vi "Gel Tugging Force Mode_Data Logger v16.20 DIC.vi"() -> ()   [LabVIEW 2015]
uses:
  <vilib>/Utility/error.llb/DialogType.ctl
  <vilib>/DAQmx/read.llb/DAQmx Read (Analog 2D DBL NChan NSamp).vi
  <vilib>/DAQmx/create/channels.llb/DAQmx Create Channel (AI-Voltage-Basic).vi
  <vilib>/DAQmx/configure/timing.llb/DAQmx Timing (Sample Clock).vi
  <vilib>/DAQmx/configure/trigger.llb/DAQmx Start Trigger (Digital Edge).vi
  <vilib>/DAQmx/miscellaneous.llb/DAQmx Fill In Error Info.vi
  <vilib>/Utility/file.llb/Write Delimited Spreadsheet (DBL).vi
  <resource>/objmgr/daqmx.rc
  <resource>/objmgr/ni.dex.rc
panel:
  in  "Filename: 2":string="R1"
  out "Loop Index":u64
  in  "Working Directory":path=path "F:/EDAC_Experiments" caption="Path"
  out "Current Plot (V)":dbl[](graph)
  out "Exposure Plot (V)":dbl[](graph)
  out "Flux Plot (V)":dbl[](graph)
  in  "Start Manual Trigger Button":bool
  in  "Trigger Type?":bool=TRUE
  in  "Notes:":string="0.75 mg/mL type I collagen gel (initial ~7.4 pH) placed in a humified incubator @ 37°C/5%CO2, Prepared on 2021-12-20\nNOT Covered with 2.6mM EDAC + 0.1M MES (pH~ 6.0) solution for 30 minutes. 1X DPBS Wash as a negative \"Treatment\"\n18-mm diameter Sylgard 184 1:10 mixture\nSylgard Mold removed after polymerization, before coating and testing.\nWashed the gel before adding the red beads with clean milliQ water\n~ 170 µL of collagen gel mix  => ~ 330 mm \n~ 350 µL of 0.09 µL M450 bead/mL was used to coat the gel until setting. Prepare as per manufacturer protocol.\n~ 350 µL of  8 µL Fluorosphere beads/mL Milli-Q water were used to coat the gel for 30 seconds\nPreconditioning of gel: at least 9 full cycles of ON/OFF with the needle tip at the start location.\nStock rat-tail type I collagen: 3.04 mg/mL. Corning. REF: 354236. Lot #:1077003\nFluoSpheres™ Carboxylate-Modified Microspheres, 0.5 µm, red fluorescent (580/605), 2% solids. REF: F8812. Lot: 2291412.\nDynabeads™ M-450 Tosylactivated 4.5 µm superparamagnetic beads containing surface tosyl groups. REF: 14013. Lot: 00789712."
  out "Total Ramp \nTime (ms)":i16
  out "# Ramp\nSteps":i16
  in  "Fluoro Beads\nDiameter (Micron)":dbl=0.5 format="%#.1g"
  in  "Tip Initial XY Separation\n (micron)":dbl=17.0
  in  "Frame Scale \n(micron/pixel)":dbl=0.24281
  in  "Gel Thickness\n(Micron)":dbl=345.0
  in  "Fluoro Beads \nZ-Level\n(Micron)":dbl
  in  "Magnetic \nBead Z-Level\n(Micron)":dbl
  in  "Tip Z-level Above Gel Surface (micron)":dbl=10.0
  out "Digital Trigger":bool
  out "Flux On\n Setpoint (Gs)":dbl=2.4945191 format="%.3g"
  out "Column 4":string="Flux Sensor (V)"
  out "Column 3":string="Flux Sensor (V)"
  out "Column 1":string="Flux Sensor (V)"
  out "Column 2":string="Flux Sensor (V)"
  in  "Temperature\n(ºC)":dbl=24.8
  out "Ready?":bool
  in  "?":bool
  in  "Relative \nHumidity (%)":dbl=22.0
  out "Magnetic Flux Sensor\n Sensitivity (V/Gs)":dbl=2.4945191 format="%#_8g"
  in  "Magnetic Bead\nDiameter (Micron)":dbl=4.5 format="%#.1g"
  in  "Needle\n Inclination \nAngle (º)":dbl=25.0
  out "Data Points":u64
  out "Cycles":i16
  out "Downloading\nData":bool
  out "Magnetic Flux Sensor\n Zero, Crude Mean (V)":dbl=2.4945191 format="%.6g"
  in  "Filename:":string="S20211220.12mm.1_0.75mgmL_37C-B1.348um-NoEDC.CO2"
  # "For Gel Tugging Experiments v16.20-DIC Part"
  # "Verify Data Further with  \"Gel Tugging Force Mode_Data Reduction v16.00.vi\" or \"ReadSensorData.m\" in MATLAB"
  # "Step 1: Enter:"
  # "-DIC-"
  # ".dat"
  # "&"
  # "_Notes.txt"
  # "Manual"
  # "Automatic"
  # "Step 2: Click TRGR or Run Macro in Nikon Elements"
  # "datapoints downloaded"
  # "out of"
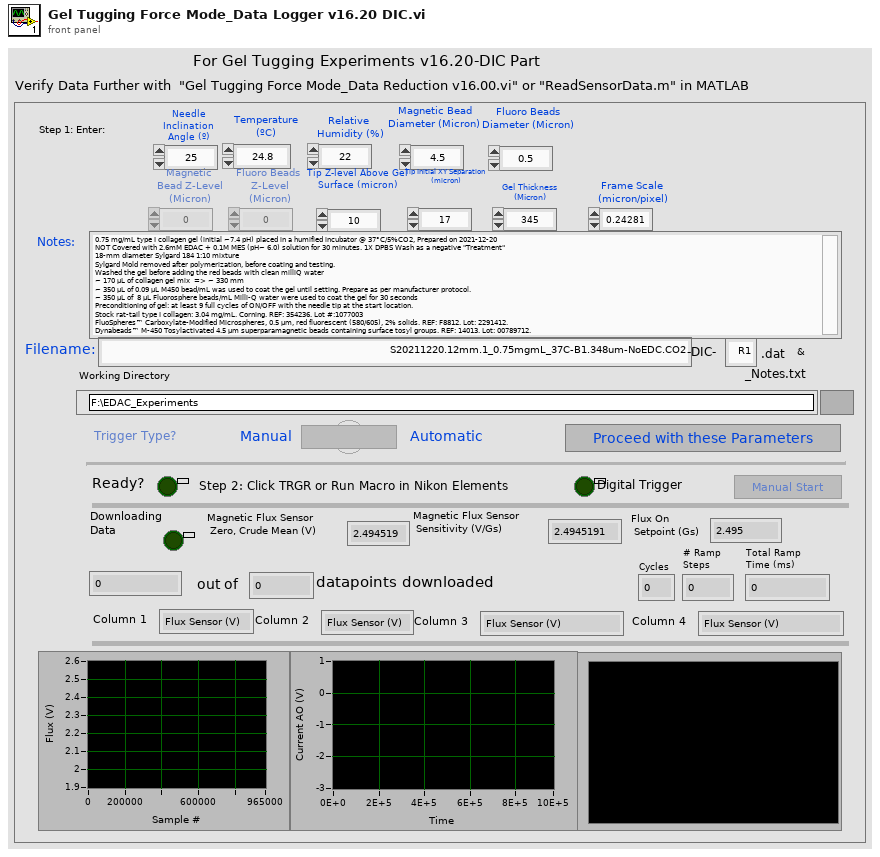
[diagram p1: front panel]
types:
  T1 = enum8{"Enabled", "Disabled", "Disabled and Grayed Out"}
  T2 = typedef "DialogType.ctl" = u16
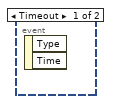
[diagram p2: hidden frame]
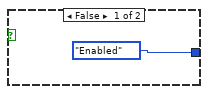
[diagram p3: hidden frame]
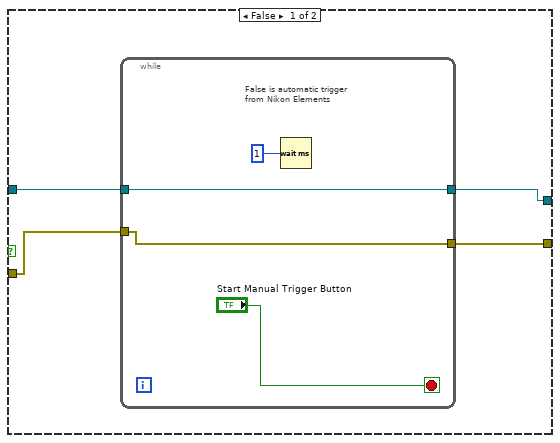
[diagram p4: hidden frame]
diagram:
  # "Modified from v15.00 by #Waddah #Moghram on 12/18/2018 and thereafter.\n1. Added a note section that will be in a file with the same note, but add \"notes\" to it. \n2. Tip -> Magnetic Bead. Magnetic Bead -> Fluorobeads. Fluoro beads -> Tip z-level. Headers were corrected 12/20/2018\n \nModified from v11.00 by #Waddah #Moghram on 5/4/2018 and thereafter:\n1. Updated the header to include gel-related information such as z-levels for the tip, bead, and thickness; gel thickness.\n2. Changed output file extension to *.dat\n3. Added a few other headers. Updated Ramp Step Information 11/28/2018\n\nModified from v10.00 by #Waddah #Moghram on 4/26/2018:\n1. This program will get the digital trigger from Nikon Elements. Then it will forward it to the control sequence VI on the slave DAQ for real-time sequence. This is a roundabout way to deal with the issue of ground loop problems.\n\nModified from v8.00 and later by #Waddah #Moghram on 4/4/2018 \n2. Just add an extra Row...with Null Flux Corrective just for the record. Did not mess with anything previously\n2. \"Flux Observed Zero\" renamed to \"Null Flux Observed\"\n3. \"AO Signal\" is replaced back to \"Camera Exposure (V)\"\n4. Added Labels \"Rows\" to the Header to keep track\n5. Updated Samples read per loop from 400 to 40000 4/1/2018\n6. Added Headers for Gel properties\n\nModified from v7.40 by #Waddah #Moghram on 1/4/2018\n1. Remove Step 0: Recording temperature with thermocouple. Thermocouple reading is not reliable, whether is the one built into labVIEW or the handheld one. Enter the value read by the Digital Thermometer along with relative humidity readings.\n2. Added an extra row to store both sets of PIDs for ON/OFF. \n3. Modified Tabbing Order on 3/4/2018\n4. Added Columns Display at front panel 3/18/2018\n\nModified from v7.30 by #Waddah #Moghram on 12/23/2017\n1. Added event close loop to make the Data Logger Running False if user closes it abruptly. \nNote: Aborting event is not included. Avoid aborting if possible.\n2. corrected total number of data points to allow for more than 2 seconds 1/4/2018 by #WIM\n\nModified from v7.00 by #Waddah #Moghram on 12/21/2017\n1. Reduce Thermocouple time to 1 \n2. Added another Text to record room temperature manual. But be consistent.\n\nModified from v6.00 by #Waddah #Moghram on 12/18/2017\n1. Added Relative Humidity Entry instead of \"Dummy Variable Entry in the Header.\" This value is to be entered from the reading of Relative Humidity\\\n2. Added Thermocouple measurement VI into this one. Average and storage into Data Logger for future purposes. \n\nModified from v5.22 by #Waddah #Moghram on 12/05/2017\n1. Added Entry for Magnetic Sensor Sensitivity\n2. Added Precisions for Header Values\n\nModified from v.4.00 by #Waddah #Moghram on 8/9/2017\n\nModified from v.3.80 by #Waddah #Moghram on 8/7/2017\n*Current Dialog boxes. Use Stacked sequences. Cleaned up v.3.80\n*Included Post  & Pre-wave Periods in Data Collection\n\nModified by #Waddah #Moghram on 8/7/2017\n*Include PID Parameters in the file\n*Modified headers of columns to be able to be extracted from MATLAB\n*Network stream loop is cleaned up \n*Removed Data Logging Time. Whatever it it takes to download the entire stream.\n*works with local single process FIFO\n\nDigital Input (Trigger)\n1. Dev3/PFI0 is connected internally in the DAQ-1/Master Connecter block. It is also wired up to DAQ-2/Slave Connector Block\n\nModifications from previous edition:\n1. Removed AI1 & AI2 to see if instability is due to a ground loop.\n\nNote: Sampling rate for Data Logger is 10,000 Samples/Second"
  n1 = flat-sequence {
    tunnel: [w18] -> w2
    tunnel: [w28] -> w12
    tunnel: [w29] -> w11
    tunnel: w2 -> [w25]
    tunnel: [w25] -> w1
    tunnel: w12 -> [w42]
    tunnel: w11 -> [w41]
    tunnel: [w43] -> w7
    tunnel: [w44] -> w3
    tunnel: w1 -> [w40]
    tunnel: [w225] -> w8
    tunnel: w7 -> [w158]
    tunnel: [w158] -> w6
    tunnel: [w288] -> w5
    tunnel: [w164] -> w4
    tunnel: w3 -> [w288]
    tunnel: w8 -> [w302]
    tunnel: w6 -> [w307]
    tunnel: [w296] -> w10
    tunnel: w5 -> [w306]
    tunnel: [w301] -> w9
    tunnel: w4 -> [w315]
    tunnel: w10 -> [w382]
    tunnel: w9 -> [w381]
    frame #0 {
      w16 = FALSE ("Data Download")
      (unwired) "1. OPEN the PID Control VI & Follow Instructions **if you have not done so already**.\n2. Click OK to begin temperature measurement & ENTER other variables afterwards.\n3. RUN the macro (if a macro is used). Otherwise, CLICK  \"TRGR\" button in Nikon Elements to initiate Fast Timelapse Image Capture, Data Acquisition, and PID-Controlled Sequence."
      # "Clear Graphs"
      # "Reset the Data Download"
      n2 = property on="Flux Plot (V)" class="WFGraph (strict)"("Value"=dbl[] [] ("Flux Plot (V)")) -> ()  [unwired: 2 in, 2 out]
      n3 = property on="Current Plot (V)" class="WFGraph (strict)"("Value"=dbl[] [] ("Current Plot (V)")) -> ()  [unwired: 2 in, 2 out]
      n4 = property on="Exposure Plot (V)" class="WFGraph (strict)"("Value"=dbl[] [] ("Exposure Plot (V)")) -> ()  [unwired: 2 in, 2 out]
      n5 = shared-variable "NI-GenericDesktopPC-3A84958E\\Kopco PS Project Target Variables Library.lvlib\\Data Download"(w16) -> ()  [unwired: 1 in, 1 out]
      n6 = shared-variable "NI-GenericDesktopPC-3A84958E\\Kopco PS Project Target Variables Library.lvlib\\Data Logger Running"(TRUE ("Data Logger Running")) -> ()  [unwired: 1 in, 1 out]
      n7 = shared-variable "NI-GenericDesktopPC-3A84958E\\Kopco PS Project Target Variables Library.lvlib\\Temperature Measured"(w16) -> ()  [unwired: 1 in, 1 out]
      n8 = shared-variable "NI-GenericDesktopPC-3A84958E\\Kopco PS Project Target Variables Library.lvlib\\Experiment Settings Entered"(w16) -> ()  [unwired: 1 in, 1 out]
      n9 = shared-variable "NI-GenericDesktopPC-3A84958E\\Kopco PS Project Target Variables Library.lvlib\\Digital Trigger"(w16) -> ()  [unwired: 1 in, 1 out]
    }
    frame #1 {
      # "Gives a pause to adjust the values before confirmation"
      # "Bound to \"Experiment Settings Entered\"\nglobal shared variable."
      n10 = while {
        tunnel: ["?"] -> w19
        tunnel: ["Trigger Type?"] -> w18
        stop <- "?" stop-if-true
        n11 = case shown="True" "Trigger Type?" {
          tunnel: [T1."Enabled" ("Disabled") T1."Disabled and Grayed Out" ("Disabled")] -> w22
          frame False {
          }
          frame True {
          }
        }
        n12 = property on="Start Manual Trigger Button" class="Bool"("Disabled"=w22) -> ()  [unwired: 2 in, 2 out]
      }
      n13 = shared-variable "NI-GenericDesktopPC-3A84958E\\Kopco PS Project Target Variables Library.lvlib\\Experiment Settings Entered"(w19) -> ()  [unwired: 1 in, 1 out]
    }
    frame #2 {
      w26 = 30000.0  # AI Frequency
      w30 = 10106 items=["Default"=-1, "RSE"=10083, "NRSE"=10078, "Differential"=10106, "Pseudodifferential"=12529] ("input terminal configuration")
      w31 = 10123 items=["Finite Samples"=10178, "Continuous Samples"=10123] ("sample mode")
      # "Configuring Analog Inputs (AIs)\n3. Dev2/AI5 is connected to \"RAW\" Magnetic Flux Sensor\n4. Dev2/AI6 is connected to \"Current Senssor (1A/V)\"\n5. Dev2/AI7 is connected to Camera Exposure Signal (\"Out 4\" on sCMOS Camera)"
      # "As of 8/3/2017. This is \njust to initiate digital trigger.\nNo data is collected via master DAQ"
      n14 = call-poly <vilib>:"DAQmx Create Virtual Channel.vi"("maximum value"=10.0, "minimum value"=-10.0, "input terminal configuration"=w30, "physical channels"="Dev3/ai3") -> ("task out"=w33:refnum<k21>, "error out"=w32:errorcluster)  [unwired: 10 in]
      n15 = call-poly <vilib>:"DAQmx Timing.vi"("task/channels in"=w33, "sample mode"=w31, "rate"=w26, "source"=tag "OnboardClock" ("Sample Clock Source"), "error in"=w32) -> ("task out"=w34:refnum<k21>, "error out"=w35:errorcluster)  [unwired: 9 in]
      n16 = call <vilib>:"DAQmx Configure Input Buffer.vi"("task/channels in"=w34, "buffer size (in samples per channel)"=200000, "error in"=w35) -> ("task out"=w28:refnum<k21>, "error out"=w29:errorcluster)  [unwired: 11 in]
    }
    frame #3 {
      n17 = case shown="True" w40 {
        tunnel: [w48 w66] -> w45
        tunnel: w41 -> [w49 w58]
        tunnel: [w51 w57] -> w46
        tunnel: w42 -> [w50 w56]
        frame False {
          n18 = while {
            tunnel: [w54] -> w51
            tunnel: w50 -> [w54]
            tunnel: w49 -> [w53]
            tunnel: [w53] -> w48
            stop <- "Start Manual Trigger Button" stop-if-true
            # "False is automatic trigger \nfrom Nikon Elements"
            n19 = Wait (ms)(milliseconds to wait=u32 1) -> ()  [unwired: 1 out]
          }
        }
        frame True {
          w59 = 10280 items=["Rising"=10280, "Falling"=10171] ("edge")
          # "True is automatic trigger \nfrom Nikon Elements"
          # "Waiting for Digital Trigger (\"TRGR\") from Nikon Element\nOr Macro that has a digital trigger"
          n20 = call-poly <vilib>:"DAQmx Trigger.vi"("task/channels in"=w56, "source"=tag "/Dev3/PFI0", "edge"=w59, "error in"=w58) -> ("task out"=w61:refnum<k21>, "error out"=w63:errorcluster)  [unwired: 10 in]
          n21 = property class="DAQmx Trigger"(reference=w61, error in=w63, "Start.DigEdge.DigFltr.MinPulseWidth"=1e-06) -> (reference out=w62:refnum<k21>, error out=w64:errorcluster)
          n22 = call <vilib>:"DAQmx Start Task.vi"("task/channels in"=w62, "error in"=w64) -> ("task out"=w57:refnum<k21>, "error out"=w66:errorcluster)  [unwired: 12 in]
        }
      }
      n23 = while "Just a one-item loop for to start the digital trigger" {
        tunnel: w45 -> [w73]
        tunnel: w46 -> [w72]
        tunnel: [w71] -> w44
        tunnel: [w70] -> w43
        tunnel: [w67] -> w47
        i -> [w69]
        stop <- w67 stop-if-true
        w75 = -1.0  # timeout
        # "Added on 4/24/2018. Digital Trigger to be transferred to \nRT control sequence VI"
        n24 = Equal?(x=1, y=w69) -> (x = y?=w67:bool)
        n25 = call-poly <vilib>:"DAQmx Read.vi"("task/channels in"=w72, "number of samples per channel"=1, "timeout"=w75, "error in"=w73) -> ("task out"=w71:refnum<k21>, "error out"=w70:errorcluster)  [unwired: 9 in, 1 out]
        n26 = Unbundle By Name(w70) -> ()  [unwired: 1 out]
      }
      n27 = shared-variable "NI-GenericDesktopPC-3A84958E\\Kopco PS Project Target Variables Library.lvlib\\Digital Trigger"(w47) -> ()  [unwired: 1 in, 1 out]
    }
    frame #4 {
      w114 = 0.0  # number
      w130 = "\t"
      w132 = "\t"
      w155 = "\t"
      w154 = "\t"
      w169 = "\t"
      w168 = "\t"
      (unwired) "AO Signal (V)" ("string")
      w189 = "\t"
      w187 = "\t"
      w215 = "\t"
      w213 = "\t"
      w274 = "\t"
      w272 = "\t"
      w240 = "\t"
      w238 = "\t"
      w175 = "Current AO (V)" ("string")
      w254 = "\t"
      w257 = "\t"
      w166 = "Camera Exposure TTL (V)" ("string")
      w251 = "\t"
      w174 = "Current Sensor (V or A)" ("string")
      w250 = "Flux Sensor (V)" ("string")
      # "Added on 3/17/2018\nfor mini DeGauss & \ntuning experiments. \nModify controller Program accordingly.\n4/4/2018. Back to Camera Exposure"
      # "Added on 3/17/2018\nfor mini DeGauss & \ntuning experiments. \nModify controller Program accordingly.\n4/4/2018. Back to Camera Exposure"
      # "Step Duration is changed to \nSampling Rate, 1/5/2018 by WIM"
      # "Sampling Rate (samples/sec)"
      # "Removed (%) on 12/20/2017 @ 6:58 PM.\nIt should not be % since it is alreayd in decimal. Otherwise, it is %"
      # "Changed from (mV/Gs) to (V/Gs) on 7/18/2017"
      # "Modified on 7/19/2017 to Including Sampling Frequency \ninstead of Sampling Rate to minimize round off Error"
      # "3rd Line Header"
      # "Magentic Sensor Sensitivity"
      n28 = shared-variable "NI-GenericDesktopPC-3A84958E\\Kopco PS Project Target Variables Library.lvlib\\Flux Setpoint ON Gs Relative"() -> (w161:dbl)  [unwired: 1 in, 1 out]
      "Flux On\n Setpoint (Gs)" <- w161
      n29 = shared-variable "NI-GenericDesktopPC-3A84958E\\Kopco PS Project Target Variables Library.lvlib\\Null Flux Pre Period"() -> (w285:dbl)  [unwired: 1 in, 1 out]
      n30 = shared-variable "NI-GenericDesktopPC-3A84958E\\Kopco PS Project Target Variables Library.lvlib\\Temperature"("Temperature\n(ºC)") -> ()  [unwired: 1 in, 1 out]
      n31 = shared-variable "NI-GenericDesktopPC-3A84958E\\Kopco PS Project Target Variables Library.lvlib\\Zero Flux Observed GS"() -> (w284:dbl)  [unwired: 1 in, 1 out]
      n32 = shared-variable "NI-GenericDesktopPC-3A84958E\\Kopco PS Project Target Variables Library.lvlib\\Null Flux Post Period"() -> (w286:dbl)  [unwired: 1 in, 1 out]
      n33 = shared-variable "NI-GenericDesktopPC-3A84958E\\Kopco PS Project Target Variables Library.lvlib\\MagneticBeadDiameterMicron"("Magnetic Bead\nDiameter (Micron)") -> ()  [unwired: 1 in, 1 out]
      n34 = shared-variable "NI-GenericDesktopPC-3A84958E\\Kopco PS Project Target Variables Library.lvlib\\PID Parameters ON"() -> (w227:dbl[])  [unwired: 1 in, 1 out]
      n35 = shared-variable "NI-GenericDesktopPC-3A84958E\\Kopco PS Project Target Variables Library.lvlib\\Sensor Sensitivity Core"() -> (w210:dbl)  [unwired: 1 in, 1 out]
      "Magnetic Flux Sensor\n Sensitivity (V/Gs)" <- w210
      n36 = shared-variable "NI-GenericDesktopPC-3A84958E\\Kopco PS Project Target Variables Library.lvlib\\NeedleInclinationAngle"("Needle\n Inclination \nAngle (º)") -> ()  [unwired: 1 in, 1 out]
      n37 = shared-variable "NI-GenericDesktopPC-3A84958E\\Kopco PS Project Target Variables Library.lvlib\\RelativeHumidity"("Relative \nHumidity (%)") -> ()  [unwired: 1 in, 1 out]
      n38 = shared-variable "NI-GenericDesktopPC-3A84958E\\Kopco PS Project Target Variables Library.lvlib\\Zero Flux Calibrated Core"() -> (w258:dbl)  [unwired: 1 in, 1 out]
      "Magnetic Flux Sensor\n Zero, Crude Mean (V)" <- w258
      n39 = Index Array(array=w227, index=3) -> (element=w287:dbl)
      n40 = Index Array(array=w227, index=4) -> (element=w164:dbl)
      n41 = Index Array(array=w227, index=2) -> (element=w231:dbl)
      n42 = Number To Fractional String "Flux ON Relative Setpoint (Gs)"(number=w161) -> (F-format string=w279:string)  [unwired: 3 in]
      n43 = Number To Fractional String "Flux Observed Zero (Gs)"(number=w284) -> (F-format string=w278:string)  [unwired: 3 in]
      n44 = Index Array(array=w227, index=1) -> (element=w234:dbl)
      n45 = Index Array(array=w227, index=0) -> (element=w236:dbl)
      n46 = Number To Fractional String "Pre- Zero Interval (s)"(number=w285) -> (F-format string=w277:string)  [unwired: 3 in]
      n47 = Number To Fractional String "Post- Zero Interval (s)"(number=w286) -> (F-format string=w273:string)  [unwired: 3 in]
      n48 = Divide(x="Relative \nHumidity (%)", y=100.0) -> (x/y=w204:dbl)
      n49 = shared-variable "NI-GenericDesktopPC-3A84958E\\Kopco PS Project Target Variables Library.lvlib\\Cycles"() -> (w270:i16)  [unwired: 1 in, 1 out]
      n50 = shared-variable "NI-GenericDesktopPC-3A84958E\\Kopco PS Project Target Variables Library.lvlib\\PID Parameters OFF"() -> (w173:dbl[])  [unwired: 1 in, 1 out]
      n51 = Number To Fractional String "Proportional Gain (K_c)"(number=w236) -> (F-format string=w246:string)  [unwired: 3 in]
      n52 = Number To Exponential String "Integral Time (T_i, min)"(number=w234) -> (E-format string=w245:string)  [unwired: 3 in]
      n53 = shared-variable "NI-GenericDesktopPC-3A84958E\\Kopco PS Project Target Variables Library.lvlib\\Needle Used"() -> (w176:i8)  [unwired: 1 in, 1 out]
      n54 = Number To Fractional String "Magnetic Sensor Mean, Crude"(number=w258, precision (6)=i16 6) -> (F-format string=w261:string)  [unwired: 2 in]
      n55 = Number To Exponential String "Derivative Time (T_d, min)"(number=w231) -> (E-format string=w244:string)  [unwired: 3 in]
      n56 = Number To Fractional String "Samples Pushed to PID at a time"(number=w287, precision (6)=i16 0) -> (F-format string=w239:string)  [unwired: 2 in]
      n57 = Number To Fractional String "Number of Cycles"(number=w270, precision (6)=i16 0 ("width (-)")) -> (F-format string=w259:string)  [unwired: 2 in]
      n58 = Number To Fractional String "Sampling Rate (Samples/Sec)"(number=w164, precision (6)=i16 0) -> (F-format string=w253:string)  [unwired: 2 in]
      n59 = Number To Fractional String "Mean Temperature (ºC)"(number="Temperature\n(ºC)", precision (6)=i16 1) -> (F-format string=w220:string)  [unwired: 2 in]
      n60 = Number To Fractional String "Inclination Angle (º)"(number="Needle\n Inclination \nAngle (º)", precision (6)=i16 0) -> (F-format string=w219:string)  [unwired: 2 in]
      n61 = Number To Fractional String "Relative Humidity (%)"(number=w204, precision (6)=i16 2 ("width (-)")) -> (F-format string=w214:string)  [unwired: 2 in]
      n62 = Number To Fractional String "Magnetic Bead Diameter (Micron)"(number="Magnetic Bead\nDiameter (Micron)", precision (6)=i16 1) -> (F-format string=w218:string)  [unwired: 2 in]
      n63 = Number To Fractional String "Magnetic Sensor Sensitivity"(number=w210, precision (6)=i16 7) -> (F-format string=w260:string)  [unwired: 2 in]
      n64 = Index Array(array=w173, index=2) -> (element=w180:dbl)
      n65 = Index Array(array=w173, index=1) -> (element=w183:dbl)
      n66 = Index Array(array=w173, index=0) -> (element=w185:dbl)
      n67 = Concatenate Strings "1st Row"("Magnetic Sensor Zero (V)" ("string"), w257, "Magnetic Sensor Sensitivity (V/Gs)" ("string"), w257, "Number of Cycles" ("string"), w257, "Sampling Rate (Samples/Sec)" ("string"), "\r") -> (w262:string)
      n68 = Number To Fractional String "OFF Proportional Gain (K_c)"(number=w185) -> (F-format string=w195:string)  [unwired: 3 in]
      n69 = Number To Exponential String "Integral Time (T_i, min)"(number=w183) -> (E-format string=w194:string)  [unwired: 3 in]
      n70 = Number To Exponential String "Derivative Time (T_d, min)"(number=w180) -> (E-format string=w193:string)  [unwired: 3 in]
      n71 = Number To Fractional String "Needle Used"(number=w176, precision (6)=i16 0) -> (F-format string=w188:string)  [unwired: 2 in]
      n72 = Concatenate Strings "2nd Row"(w262, w261, w254, w260, w254, w259, w254, w253, "\r") -> (w230:string)
      n73 = Concatenate Strings "3rd Row"(w230, "ON Proportional Gain (K_c)" ("string"), w238, " Integral Time (T_i, min)" ("string"), w238, "Derivative Time (T_d, min)" ("string"), w238, "Samples pushed to PID" ("string"), "\r") -> (w247:string)
      n74 = Concatenate Strings "4th Row"(w247, w246, w240, w245, w240, w244, w240, w239, "\r") -> (w178:string)
      n75 = Concatenate Strings "5th Row"(w178, "OFF Proportional Gain (K_c)" ("string"), w187, "Integral Time (T_i, min)" ("string"), w187, "Derivative Time (T_d, min)" ("string"), w187, "Needle Used" ("string"), "\r") -> (w196:string)
      n76 = shared-variable "NI-GenericDesktopPC-3A84958E\\Kopco PS Project Target Variables Library.lvlib\\Zero Flux Observed Gs Corrected"() -> (w162:dbl)  [unwired: 1 in, 1 out]
      n77 = shared-variable "NI-GenericDesktopPC-3A84958E\\Kopco PS Project Target Variables Library.lvlib\\TipZaboveGelMicron"("Tip Z-level Above Gel Surface (micron)") -> ()  [unwired: 1 in, 1 out]
      n78 = shared-variable "NI-GenericDesktopPC-3A84958E\\Kopco PS Project Target Variables Library.lvlib\\TipBeadXYSeparationMicron"("Tip Initial XY Separation\n (micron)") -> ()  [unwired: 1 in, 1 out]
      n79 = Concatenate Strings "6th Row"(w196, w195, w189, w194, w189, w193, w189, w188, "\r") -> (w177:string)
      n80 = Concatenate Strings "7th Row"(w177, "Flux ON Relative Setpoint (Gs)" ("string"), w272, "Null Flux - Observed (Gs)" ("string"), w272, "Pre-Zero Interval (s)" ("string"), w272, "Post-Zero Interval (s)" ("string"), "\r") -> (w280:string)
      n81 = Concatenate Strings "8th Row"(w280, w279, w274, w278, w274, w277, w274, w273, "\r") -> (w211:string)
      n82 = Concatenate Strings "9th Row"(w211, "Temperature (ºC)" ("string"), w213, "Needle Inclination Angle (º)" ("string"), w213, "Magnetic Beads Diameter (Micron)" ("string"), w213, "Relative Humidity" ("string"), "\r") -> (w221:string)
      n83 = Concatenate Strings "10th Row"(w221, w220, w215, w219, w215, w218, w215, w214, "\r") -> (w165:string)
      n84 = Concatenate Strings "11th Row"(w165, "Null Flux Corrected (Gs)" ("string"), w168, "=====================" ("string"), w168, "=====================" ("string"), w168, "Tip Z-level Above Gel Surface (Micron)" ("string"), "\r") -> (w163:string)
      n85 = Number To Fractional String "Mag bead\n Z-Level\n(Micron)"(number="Magnetic \nBead Z-Level\n(Micron)", precision (6)=i16 2) -> (F-format string=w136:string)  [unwired: 2 in]
      n86 = Number To Fractional String "Tip Z-Level\n(Micron)"(number="Tip Z-level Above Gel Surface (micron)", precision (6)=i16 2) -> (F-format string=w134:string)  [unwired: 2 in]
      n87 = Number To Fractional String "Fluoro Z-Level\n(Micron)"(number="Fluoro Beads \nZ-Level\n(Micron)", precision (6)=i16 2) -> (F-format string=w135:string)  [unwired: 2 in]
      n88 = Number To Fractional String "Null Flux Corrected (GS)"(number=w162) -> (F-format string=w172:string)  [unwired: 3 in]
      n89 = shared-variable "NI-GenericDesktopPC-3A84958E\\Kopco PS Project Target Variables Library.lvlib\\Ramp Total Interval (ms)"() -> (w113:dbl)  [unwired: 1 in, 1 out]
      "Total Ramp \nTime (ms)" <- w113
      n90 = shared-variable "NI-GenericDesktopPC-3A84958E\\Kopco PS Project Target Variables Library.lvlib\\FrameScaleMicronPerPixel"("Frame Scale \n(micron/pixel)") -> ()  [unwired: 1 in, 1 out]
      n91 = shared-variable "NI-GenericDesktopPC-3A84958E\\Kopco PS Project Target Variables Library.lvlib\\Ramp Steps"() -> (w112:i16)  [unwired: 1 in, 1 out]
      "# Ramp\nSteps" <- w112
      n92 = Concatenate Strings "12th Row"(w163, w172, w169, w136, w169, w135, w169, w134, "\r") -> (w151:string)
      n93 = Concatenate Strings "13th Row"(w151, "Gel Thickness (Micron)" ("string"), w154, "Tip Initial XY Separation (micron)" ("string"), w154, "Frame Scale (micron/pixel)" ("string"), w154, "Fluoro Beads Diameter (Micron)" ("string"), "\r") -> (w152:string)
      n94 = Number To Fractional String "Image Scale\n (micron/pixel)"(number="Frame Scale \n(micron/pixel)", precision (6)=i16 5) -> (F-format string=w149:string)  [unwired: 2 in]
      n95 = shared-variable "NI-GenericDesktopPC-3A84958E\\Kopco PS Project Target Variables Library.lvlib\\FluorescentMicrospheresDiameterMicron"("Fluoro Beads\nDiameter (Micron)") -> ()  [unwired: 1 in, 1 out]
      n96 = Number To Fractional String "Initial Separation\nDistance (micron)"(number="Tip Initial XY Separation\n (micron)", precision (6)=i16 2) -> (F-format string=w148:string)  [unwired: 2 in]
      n97 = Number To Fractional String(number=w112, precision (6)=i16 0) -> (F-format string=w122:string)  [unwired: 2 in]
      n98 = Number To Fractional String(number=w113, precision (6)=i16 0) -> (F-format string=w121:string)  [unwired: 2 in]
      n99 = Number To Fractional String(number=w114, precision (6)=i16 1) -> (F-format string=w120:string)  [unwired: 2 in]
      n100 = Number To Fractional String(number=w114, precision (6)=i16 1) -> (F-format string=w119:string)  [unwired: 2 in]
      n101 = shared-variable "NI-GenericDesktopPC-3A84958E\\Kopco PS Project Target Variables Library.lvlib\\GelThicknessMicron"("Gel Thickness\n(Micron)") -> ()  [unwired: 1 in, 1 out]
      n102 = Number To Fractional String "Gel Measured Thickness (Micron)"(number="Gel Thickness\n(Micron)", precision (6)=i16 2) -> (F-format string=w147:string)  [unwired: 2 in]
      n103 = Number To Fractional String "Fluoro Beads Diameter (Micron)"(number="Fluoro Beads\nDiameter (Micron)", precision (6)=i16 1) -> (F-format string=w150:string)  [unwired: 2 in]
      n104 = Concatenate Strings("Filename:", "-DIC-" ("string"), "Filename: 2") -> (w85:string)
      n105 = Path To String(path="Working Directory") -> (string=w81:string)
      n106 = Concatenate Strings "14th Row"(w152, w147, w155, w148, w155, w149, w155, w150, "\r") -> (w125:string)
      n107 = Concatenate Strings "15th Row"(w125, "Ramp Steps" ("string"), w130, "Total Ramp Time (ms)" ("string"), w130, "===============" ("string"), w130, "===============" ("string"), "\r") -> (w124:string)
      n108 = shared-variable "NI-GenericDesktopPC-3A84958E\\Kopco PS Project Target Variables Library.lvlib\\DataFileName"("Filename:") -> ()  [unwired: 1 in, 1 out]
      n109 = Concatenate Strings "16th Row"(w124, w122, w132, w121, w132, w120, w132, w119, "\r") -> (w123:string)
      n110 = shared-variable "NI-GenericDesktopPC-3A84958E\\Kopco PS Project Target Variables Library.lvlib\\DataFolderName"(w81) -> ()  [unwired: 1 in, 1 out]
      n111 = Concatenate Strings(w85, "_Notes") -> (w108:string)
      n112 = Concatenate Strings "note file name"(w108, ".txt" ("string")) -> (w79:string)
      n113 = Concatenate Strings "data file name"(w85, ".dat") -> (w80:string)
      n114 = Get Date/Time String() -> (date string=w104:string, time string=w102:string)  [unwired: 3 in]
      n115 = Build Path(base path="Working Directory", name or relative path=w80) -> (appended path=w82:path)
      n116 = Concatenate Strings "Notes\nData Header"("Notes for \"", w80, "\" collected on " ("string"), w104, " at " ("string"), w102, ":" ("string"), "\r", "Notes:") -> (w101:string)
      n117 = shared-variable "NI-GenericDesktopPC-3A84958E\\Kopco PS Project Target Variables Library.lvlib\\Notes"("Notes:") -> ()  [unwired: 1 in, 1 out]
      n118 = Build Path(base path="Working Directory", name or relative path=w79) -> (appended path=w77:path)
      n119 = Write to Text File(file (use dialog)=w77, text=w101) -> (refnum out=w111:refnum<file>, error out=w110:errorcluster)  [unwired: 2 in, 1 out]
      n120 = Concatenate Strings "17th Row\nData Header"(w123, w175, w251, w250, w251, w174, w251, w166, "\r") -> (w266:string)
      n121 = Close File(refnum=w111, error in=w110) -> ()  [unwired: 2 out]
      n122 = Write to Text File(file (use dialog)=w82, text=w266) -> (refnum out=w267:refnum<file>, error out=w268:errorcluster)  [unwired: 2 in, 1 out]
      n123 = Close File(refnum=w267, error in=w268) -> (path=w225:path)  [unwired: 1 out]
      "Column 2" <- w250
      "Column 1" <- w175
      "Column 3" <- w174
      "Column 4" <- w166
    }
    frame #5 {
      w290 = 4.0  # 4 columns
      w303 = 40000  # Samples Read per loop
      # "100000000 from 36000000 on 3/31/2018"
      # "For 2 minutes"
      # "Note: Each Step is a second"
      # "Sampling Rate (Samples per second)"
      # "I.P. Address of\nRemote Desktop"
      n124 = shared-variable "NI-GenericDesktopPC-3A84958E\\Kopco PS Project Target Variables Library.lvlib\\Period Per Cycle"() -> (w308:dbl)  [unwired: 1 in, 1 out]
      n125 = shared-variable "NI-GenericDesktopPC-3A84958E\\Kopco PS Project Target Variables Library.lvlib\\Null Flux Post Period"() -> (w313:dbl)  [unwired: 1 in, 1 out]
      n126 = shared-variable "NI-GenericDesktopPC-3A84958E\\Kopco PS Project Target Variables Library.lvlib\\Null Flux Pre Period"() -> (w314:dbl)  [unwired: 1 in, 1 out]
      n127 = shared-variable "NI-GenericDesktopPC-3A84958E\\Kopco PS Project Target Variables Library.lvlib\\Cycles"() -> (w309:i16)  [unwired: 1 in, 1 out]
      "Cycles" <- w309
      n128 = Multiply "Total Cycles (s)"(x=w309, y=w308) -> (x*y=w311:dbl)
      n129 = Add "Pre&Post (s)"(x=w314, y=w313) -> (x+y=w310:dbl)
      n130 = shared-variable "NI-GenericDesktopPC-3A84958E\\Kopco PS Project Target Variables Library.lvlib\\Samples Total"() -> (w289:u64)  [unwired: 1 in, 1 out]
      "Data Points" <- w289
      n131 = Add "Total Time\n(s)"(x=w311, y=w310) -> (x+y=w312:dbl)
      n132 = Multiply "Samples per column"(x=w312, y=w315) -> ()  [unwired: 1 out]
      n133 = Multiply "Total # of \nSamples"(x=w290, y=w289) -> (x*y=w291:dbl)
      n134 = Divide "Number of Loops"(x=w291, y=w303) -> (x/y=w292:dbl)
      n135 = Create Network Stream Reader Endpoint(7:100000000 ("reader buffer size"), 9:0.0 ("Double"), 10:"//169.254.136.220/FluxWriter" ("writer url"), 11:"FluxReader" ("reader name")) -> (0:w304:errorcluster, 3:w305:refnum<k21>)  [unwired: 3 in]
      n136 = while {
        tunnel: w305 -> [w365]
        tunnel: w304 -> [w364]
        tunnel: [w329] -> w299
        tunnel: [w363] -> w300
        tunnel: w302 -> [w360]
        tunnel: w307 -> [w366]
        tunnel: [w366] -> w297
        tunnel: w292 -> [_]
        tunnel: w306 -> [w352]
        tunnel: [w352] -> w301
        shift-right: [w337] -> w298
        shift-left: dbl[] [] -> [w347]
        shift-right: [w330] -> w293
        shift-left: dbl[] [] -> [w344]
        tunnel: w303 -> [w335]
        tunnel: w291 -> [_]
        tunnel: w290 -> [w327]
        tunnel: w289 -> [w326]
        i -> [w328]
        stop <- w324 stop-if-true
        w338 = 90000  # y
        # "Error 314220 is \nsometimes caused, \nbut all the data should\nbe available once the \nstream is flushed on the other side"
        # "Bound to \"Data Download\""
        # "Delete First 0's from Network Stream"
        # "Offset by Samples Taken Per loop to stop at exactly the right amount of samples\nThe last dialog box is invisible for whatever reason. To find it, Search (CTRL+F) \"TRGR\", and then \nclick \"GO TO\" the first choice. Type an arrow key. 8/8/2017"
        n137 = shared-variable-read ("Read Multiple Elements from Stream")(w365, w364, w335) -> (w329:refnum<k21>, w363:errorcluster, w359:dbl[])  [unwired: 1 in, 1 out]
        n138 = Decimate 1D Array "Input is interleaved"(w359) -> (w358:dbl[], w351:dbl[], w357:dbl[], w350:dbl[])
        n139 = property class="Network Stream Endpoint"(reference=w329) -> ("TotalElmntsWritten"=w325:u64)  [unwired: 1 in, 2 out]
        n140 = Equal?(x=0, y=w328) -> (x = y?=w354:bool)
        n141 = Build Array(w358, w351, w357, w350) -> (w353:dbl[][])
        n142 = Transpose 2D Array(2D array=w353) -> (transposed array=w355:dbl[][])
        n143 = case shown="True" w354 {
          tunnel: w355 -> [w374 w376]
          tunnel: [w374 w375] -> w349
          frame False {
          }
          frame True {
            n144 = Delete From Array(array=w376, length=1, index (row)=0) -> (array with subset deleted=w375:dbl[][])  [unwired: 1 in, 1 out]
          }
        }
        n145 = Quotient & Remainder(x=w325, y=w327) -> (floor(x/y)=w323:dbl)  [unwired: 1 out]
        n146 = Decrement(x=w323) -> (x-1=w322:dbl)
        "Loop Index" <- w322
        n147 = Greater Or Equal?(x=w322, y=w326) -> (x >= y?=w324:bool)
        n148 = Transpose 2D Array(2D array=w349) -> (transposed array=w341:dbl[][])
        n149 = call-poly <vilib>:"Write Delimited Spreadsheet.vi"("file path (dialog if empty)"=w360, "format (%.3f)"="%#.6g", "2D data"=w349, "append to file? (F)"=TRUE) -> ()  [unwired: 10 in, 2 out]
        n150 = Delete From Array(array=w341, index (row)=1 ("index")) -> (deleted portion=w348:dbl[])  [unwired: 2 in, 1 out]
        n151 = Delete From Array(array=w341, index (row)=2 ("index")) -> (deleted portion=w345:dbl[])  [unwired: 2 in, 1 out]
        n152 = Delete From Array(array=w341, index (row)=3 ("index")) -> (deleted portion=→"Exposure Plot (V)":dbl[])  [unwired: 2 in, 1 out]
        n153 = Build Array (concatenate)(w347, w348) -> (w333:dbl[])
        n154 = Build Array (concatenate)(w344, w345) -> (w332:dbl[])
        n155 = Not(x=w324) -> (.not. x?=w321:bool)
        n156 = Array Size(array=w332) -> (size(s)=w340:i32)
        n157 = Less?(x=w340, y=w338) -> (x < y?=w339:bool)
        n158 = Multiply(x=2, y=w335) -> (x*y=w336:i32)
        n159 = case shown="True" w339 {
          tunnel: [w368 w369] -> w330
          tunnel: w332 -> [w368 w373]
          tunnel: w333 -> [w367 w372]
          tunnel: [w367 w370] -> w337
          tunnel: w336 -> [_ w371]
          frame False {
          }
          frame True {
            n160 = Delete From Array(array=w373, length=w371) -> (deleted portion=w369:dbl[])  [unwired: 1 in, 1 out]
            n161 = Delete From Array(array=w372, length=w371) -> (deleted portion=w370:dbl[])  [unwired: 1 in, 1 out]
          }
        }
        n162 = shared-variable "NI-GenericDesktopPC-3A84958E\\Kopco PS Project Target Variables Library.lvlib\\Data Download"(w321) -> ()  [unwired: 1 in, 1 out]
      }
      "Flux Plot (V)" <- w298
      "Current Plot (V)" <- w293
      n163 = Destroy Stream Endpoint(8:w300, 11:w299) -> (0:w320:errorcluster)
      n164 = Merge Errors(w297, w320) -> (w296:errorcluster)
    }
    frame #6 {
      w380 = FALSE ("Data Logger Running")
      w386 = T2 3 items=["no dialog", "OK message", "continue or stop message", "OK message + warnings", "continue/stop + warnings"] ("type of dialog (OK msg:1)")
      n165 = call <vilib>:"DAQmx Stop Task.vi"("task/channels in"=w381, "error in"=w382) -> ("task out"=w385:refnum<k21>, "error out"=w384:errorcluster)  [unwired: 12 in]
      n166 = shared-variable "NI-GenericDesktopPC-3A84958E\\Kopco PS Project Target Variables Library.lvlib\\Temperature Measured"(w380) -> ()  [unwired: 1 in, 1 out]
      n167 = shared-variable "NI-GenericDesktopPC-3A84958E\\Kopco PS Project Target Variables Library.lvlib\\Experiment Settings Entered"(w380) -> ()  [unwired: 1 in, 1 out]
      n168 = shared-variable "NI-GenericDesktopPC-3A84958E\\Kopco PS Project Target Variables Library.lvlib\\Digital Trigger"(w380) -> ()  [unwired: 1 in, 1 out]
      n169 = shared-variable "NI-GenericDesktopPC-3A84958E\\Kopco PS Project Target Variables Library.lvlib\\Data Logger Running"(w380) -> ()  [unwired: 1 in, 1 out]
      n170 = shared-variable "NI-GenericDesktopPC-3A84958E\\Kopco PS Project Target Variables Library.lvlib\\Data Upload"(FALSE ("Data Upload")) -> ()  [unwired: 1 in, 1 out]
      n171 = call <vilib>:"DAQmx Clear Task.vi"("task in"=w385, "error in"=w384) -> ("error out"=w383:errorcluster)  [unwired: 13 in]
      n172 = call <vilib>:"Simple Error Handler.vi"("type of dialog (OK msg:1)"=w386, "error in (no error)"=w383) -> ()  [unwired: 3 in, 5 out]
    }
    frame #7 {
      (unwired) "OK!"
      (unwired) "1. TURN OFF \"TRGR\" if clicked inside Nikon Elements\n2. VERIFY that the \"Number of Data Points\" matches the number displayed in the \"Gel Tugging Force Mode_Data Reduction v16.00.vi\"  (It should be one sample more than the latest index)."
    }
    frame #8 {
      n173 = Stop() -> ()  [unwired: 1 in]
    }
  }
  n174 = event shown="[1] Panel Close?" {
    selector: _ -> [_ _]
    dyn-events: _ -> [_ _]
    timeout: _ -> [_ _]
    event Timeout {
      n175 = event-data() -> ()  [unwired: 1 in, 2 out]
    }
    event Panel Close? {
      n176 = event-data() -> ()  [unwired: 1 in, 3 out]
      n177 = shared-variable "NI-GenericDesktopPC-3A84958E\\Kopco PS Project Target Variables Library.lvlib\\Data Logger Running"(FALSE ("Data Logger Running")) -> ()  [unwired: 1 in, 1 out]
      n178 = event-data() -> ()  [unwired: 2 in, 1 out]
    }
  }
